vi "glyph_yellow.vi"() -> (1 "image data":T1)   [LabVIEW 2015]
uses:
  <vilib>/picture/picture.llb/imagedata.ctl
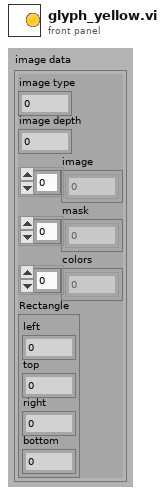
[diagram p1: front panel]
types:
  T1 = typedef "imagedata.ctl" = cluster{"image type":i32, "image depth":i32, "image":u8[], "mask":u8[], "colors":u32[], "Rectangle":cluster{"left":i16, "top":i16, "right":i16, "bottom":i16}}
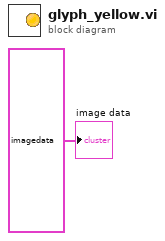
[diagram p0: block diagram]
diagram:
  "image data" <- T1 {"image type"=0, "image depth"=32, "image"=array[1024 elements], "mask"=[0, 0, 15, 224, 31, 248, 63, 252, 127, 252, 127, 254, 127, 254, 127, 254, 127, 254, 127, 254, 127, 254, 63, 252, 63, 252, 31, 248, 7, 224, 0, 0], "colors"=[], "Rectangle"={"left"=0, "top"=0, "right"=16, "bottom"=16}} ("image data")
